vi "New Int64Array DVR.vi"(8 "error in (no error)":errorcluster, 11 "Int64Array in":refnum<class "Int64Array.lvclass">) -> (0 "error out":errorcluster, 3 "Int64Array DVR out":refnum<data-value>)   [LabVIEW 2015, in "MDSplus.lvlib" / "Int64Array.lvclass"]
uses:
  <vilib>/MDSplus/Classes/Data_Class/Array_Class/Int64Array_Class/Int64Array.lvclass
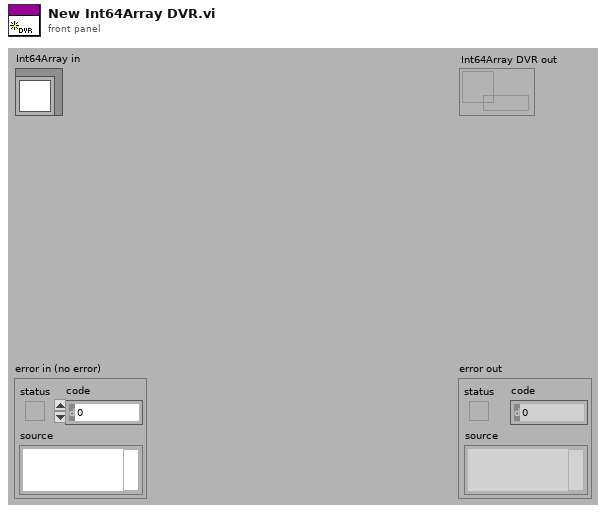
[diagram p1: front panel]
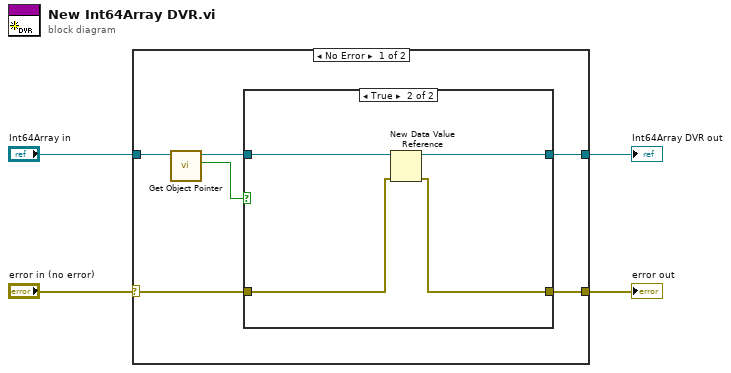
[diagram p0: block diagram]
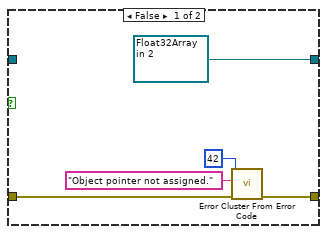
[diagram p2: hidden frame]
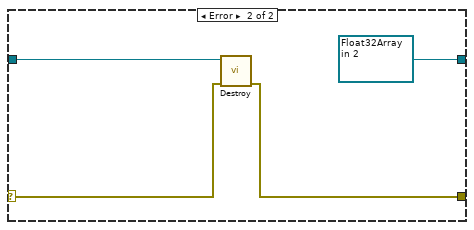
[diagram p3: hidden frame]
diagram:
  n1 = case shown="No Error" "error in (no error)" {
    selector: "error in (no error)" -> [w5 w22]
    tunnel: [w10 w21] -> w4
    tunnel: [w9 refnum<data-value> refnum ("data value reference")] -> w3
    tunnel: "Int64Array in" -> [w8 w23]
    frame No Error {
      n2 = call-dynamic "Get Object Pointer.vi"("Data in"=w8) -> ("Assigned object pointer?"=w6:bool, "Data out"=w7:refnum<class "Int64Array.lvclass">)  [unwired: 8 in, 1 out]
      n3 = case shown="True" w6 {
        tunnel: w5 -> [w12 w19]
        tunnel: [w11 w16] -> w10
        tunnel: w7 -> [_ w18]
        tunnel: [refnum<data-value> refnum ("data value reference") w17] -> w9
        frame False {
          n4 = call <vilib>:"Error Cluster From Error Code.vi"("error in (no error)"=w12, "error message (\"\")"="Object pointer not assigned." ("error message (\"\")"), "error code (0)"=42) -> ("error out"=w11:errorcluster)  [unwired: 6 in]
        }
        frame True {
          n5 = New Data Value Reference(data value=w18, error in=w19) -> (data value reference=w17:refnum<data-value>, error out=w16:errorcluster)
        }
      }
    }
    frame Error {
      n6 = call-dynamic "Destroy.vi"("error in (no error)"=w22, "Int64Array in"=w23) -> ("error out"=w21:errorcluster)  [unwired: 9 in]
    }
  }
  "error out" <- w4
  "Int64Array DVR out" <- w3
